vi "FiberSpectrograph_issueCommand_setLogLevel.vi"(8 "error in (no error)":errorcluster, 11 "command_setLogLevel_Ctl":T1) -> (0 "error out":errorcluster, 2 "function return":i32, 3 "command_setLogLevel_Ctl out":T1)   [LabVIEW 2016, in "SALLV_FiberSpectrograph.lvlib"]
doc: "int FiberSpectrograph_shm_issueCommand_setLogLevelLV(FiberSpectrograph_command_setLogLevelLV *command_setLogLevel_Ctl );"
uses:
  SALLV_FiberSpectrograph.lvlib
  DataTypes/command_setLogLevel.ctl
  SALLV_FiberSpectrograph.so
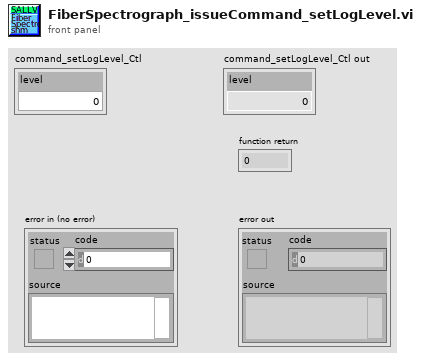
[diagram p1: front panel]
types:
  T1 = typedef "SALLV_FiberSpectrograph.lvlib/command_setLogLevel.ctl" = cluster{"level":i32}
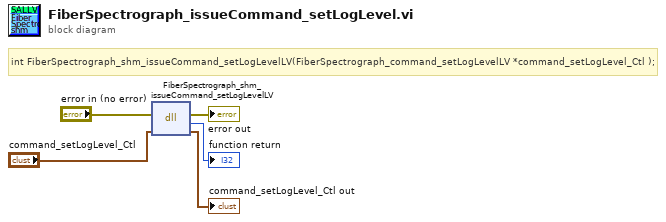
[diagram p0: block diagram]
diagram:
  # "int FiberSpectrograph_shm_issueCommand_setLogLevelLV(FiberSpectrograph_command_setLogLevelLV *command_setLogLevel_Ctl );"
  n1 = dll-call lib="home/harini/Documents/lsst/SALLV_FiberSpectrograph/SALLV_FiberSpectrograph.*" fn="FiberSpectrograph_shm_issueCommand_setLogLevelLV"(error in="error in (no error)", "command_setLogLevel_Ctl"="command_setLogLevel_Ctl") -> (error out=→"error out":errorcluster, →"function return":i32, "command_setLogLevel_Ctl"=→"command_setLogLevel_Ctl out":T1)  [unwired: 2 in, 1 out]
